vi "feedback-negative.vi"(7 "callee":refnum<vi>, 8 "error in (no error)":errorcluster, 10 "process_error":errorcluster, 11 "dialog_text":string) -> (0 "error out":errorcluster)   [LabVIEW 2015, in "lv-dialog.lvlib"]
uses:
  lv-dialog.lvlib
  api/v1/public/class/v1.lvclass
  api/v1/v1.lvlib
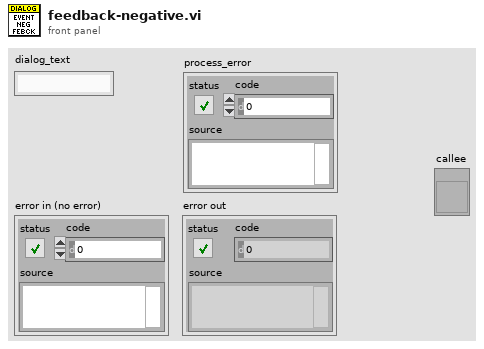
[diagram p1: front panel]
types:
  T1 = cluster{"dialog_text":string, "boolean_text_1":string, "boolean_text_2":string}
  T2 = typedef "lv-dialog.lvlib/v1.lvlib/dialog_selection.ctl" = enum16{"null", "panel_closed", "button_1", "button_2", "button_3", "cancelled"}
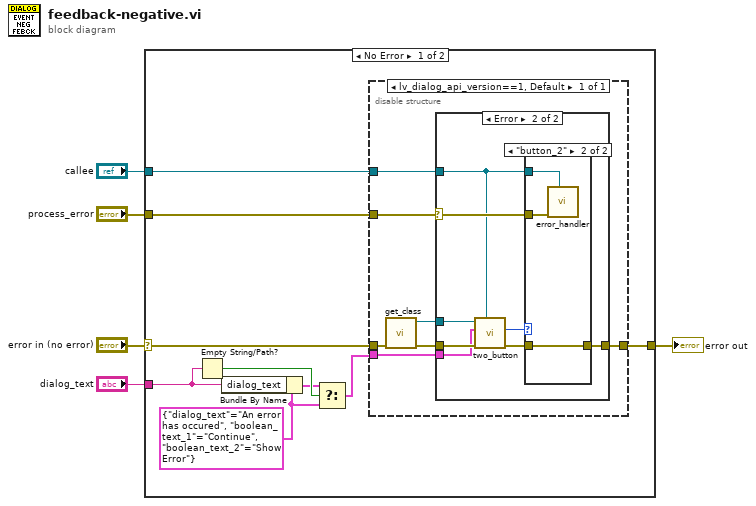
[diagram p0: block diagram]
diagram:
  n1 = case shown="No Error" "error in (no error)" {
    selector: "error in (no error)" -> [w9 w35]
    tunnel: "callee" -> [w14 _]
    tunnel: [w11 w35] -> w4
    tunnel: "process_error" -> [w10 _]
    tunnel: "dialog_text" -> [w8 _]
    frame No Error {
      w6 = T1 {"dialog_text"="An error has occured", "boolean_text_1"="Continue", "boolean_text_2"="Show Error"} ("configuration")
      n2 = Empty String/Path?(string/path=w8) -> (empty?=w13:bool)
      n3 = Bundle By Name(cluster=w6, "dialog_text"=w8) -> (w7:T1)
      n4 = Select(t=w7, s=w13, f=w6) -> (s? t:f=w12:T1)
      n5 = disable-structure shown="lv_dialog_api_version==1, Default" {
        disable-tunnel: w14 -> [w21]
        disable-tunnel: w12 -> [w20]
        disable-tunnel: [w19] -> w11
        disable-tunnel: w10 -> [w18]
        disable-tunnel: w9 -> [w17]
        frame condition #0 (active) {
          n6 = call "get_class.vi"("error in (no error)"=w17) -> ("error out"=w16:errorcluster, "class"=w15:refnum<class "v1.lvclass">)  [unwired: 9 in]
          n7 = case shown="Error" w18 {
            selector: w18 -> [_ w27]
            tunnel: w21 -> [_ w25]
            tunnel: w20 -> [_ w23]
            tunnel: [w22 w28] -> w19
            tunnel: w16 -> [w22 w26]
            tunnel: w15 -> [_ w24]
            frame No Error {
            }
            frame Error {
              n8 = call-dynamic "two_button.vi"("callee"=w25, "error in (no error)"=w26, "configuration"=w23, "v1 in"=w24) -> ("error out"=w29:errorcluster, "dialog_selection"=w30:T2)  [unwired: 5 in, 1 out]
              n9 = case shown="\"button_2\"" w30 {
                tunnel: w27 -> [_ w32]
                tunnel: w29 -> [w31 w34]
                tunnel: [w31 w34] -> w28
                tunnel: w25 -> [_ w33]
                frame Default {
                }
                frame "button_2" {
                  n10 = call "error_handler.vi"("calling_vi"=w33, "error in (no error)"=w32) -> ()  [unwired: 9 in, 1 out]
                }
              }
            }
          }
        }
      }
    }
    frame Error {
    }
  }
  "error out" <- w4
